vi "powerdelivery reset Power Data Object To Default.vi"(6 "ruleIndex":u8, 7 "powerRole":u8, 8 "error in (no error)":errorcluster, 9 "index":i32, 10 "result":cluster{"value":i32, "error":i32}, 11 "id":u32) -> (0 "error out":errorcluster, 2 "result out":cluster{"value":i32, "error":i32}, 3 "id out":u32)   [LabVIEW 2014, in "BrainStem2_LabVIEW_Library.lvlib"]
doc: "aLIBEXPORT void __stdcall powerdelivery_resetPowerDataObjectToDefault ( unsigned int* id, struct Result* result, const int index , const unsigned char powerRole , const unsigned char ruleIndex ) ;"
uses:
  BrainStem2_LabVIEW_Library.lvlib
  BrainStem2_LabVIEW.dll
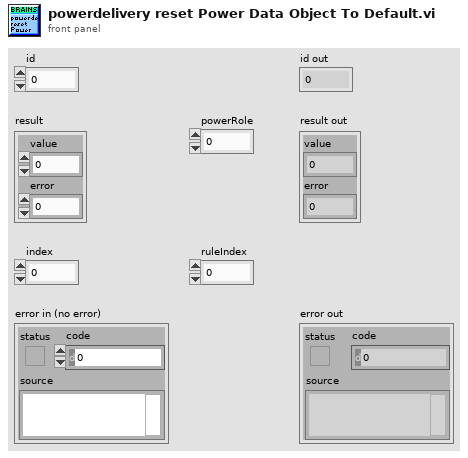
[diagram p1: front panel]
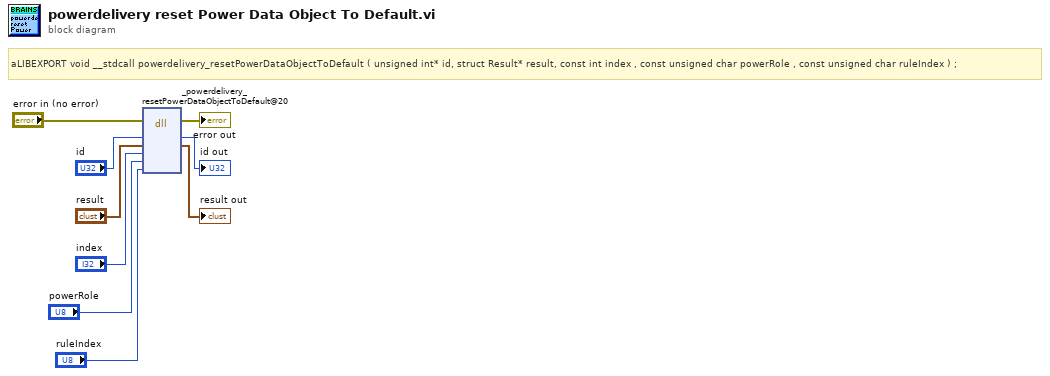
[diagram p0: block diagram]
diagram:
  # "aLIBEXPORT void __stdcall powerdelivery_resetPowerDataObjectToDefault ( unsigned int* id, struct Result* result, const int index , const unsigned char powerRole , const unsigned char ruleIndex ) ;"
  n1 = dll-call lib="C:/Users/mitch/Documents/development/acroname/software/acroname/aSource/BrainStem2/BrainStem2_LabVIEW/LabVIEW_2014_Distribution/BrainStem2_LabVIEW_w32/BrainStem2_LabVIEW.*" fn="_powerdelivery_resetPowerDataObjectToDefault@20"(error in="error in (no error)", "id"="id", "result"="result", "index"="index", "powerRole"="powerRole", "ruleIndex"="ruleIndex") -> (error out=→"error out":errorcluster, "id"=→"id out":u32, "result"=→"result out":cluster{"value":i32, "error":i32})  [unwired: 6 in, 1 out]
